vi "GDSProject_GetFullItemName.vi"(4 "error in (no error)":errorcluster, 7 "ProjectItem Refnum":refnum<vi>) -> (0 "error out":errorcluster, 3 "ItemFullName":string)   [LabVIEW 2020]
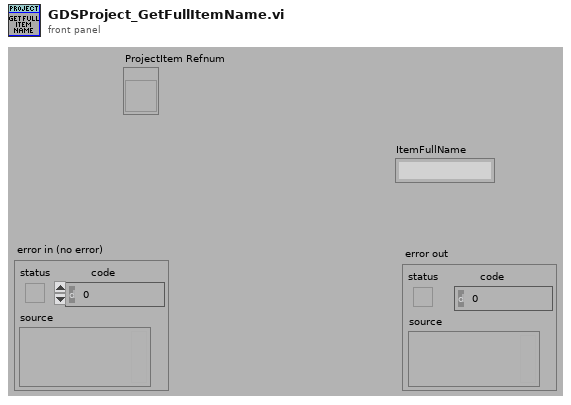
[diagram p1: front panel]
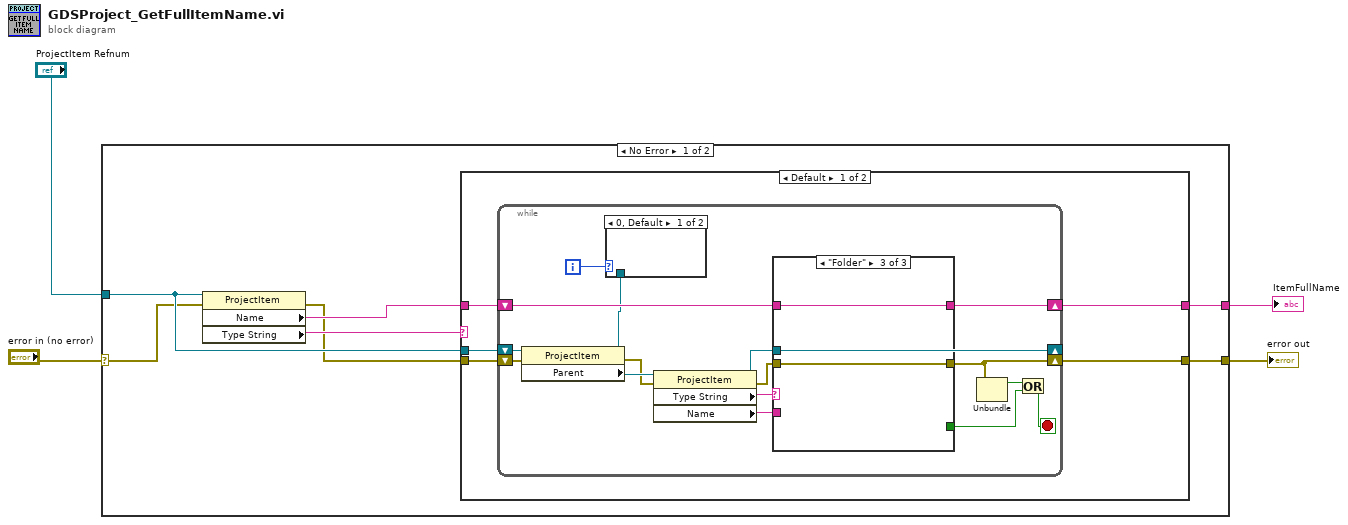
[diagram p0: block diagram]
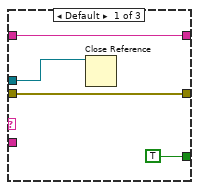
[diagram p2: hidden frame]
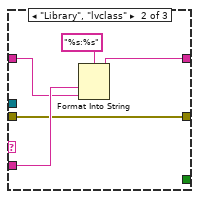
[diagram p3: hidden frame]
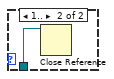
[diagram p4: hidden frame]
diagram:
  n1 = case shown="No Error" "error in (no error)" {
    selector: "error in (no error)" -> [w6 w46]
    tunnel: [w8 w46] -> w2
    tunnel: "ProjectItem Refnum" -> [w11 _]
    tunnel: [w7 _] -> w1
    frame No Error {
      n2 = property class="ProjectItem"(reference=w11, error in=w6) -> (error out=w5:errorcluster, "Name"=w9:string, "Type String"=w10:string)  [unwired: 1 out]
      n3 = case shown="Default" w10 {
        tunnel: w11 -> [w16 _]
        tunnel: w9 -> [w15 _]
        tunnel: w5 -> [w14 w45]
        tunnel: [w13 w45] -> w8
        tunnel: [w12 _] -> w7
        frame Default {
          n4 = while {
            shift-right: [w17] -> _
            shift-left: w16 -> [w32]
            shift-right: [w20] -> w12
            shift-left: w15 -> [w21]
            shift-right: [w26] -> w13
            shift-left: w14 -> [w27]
            i -> [w31]
            stop <- w23 stop-if-true
            n5 = property class="ProjectItem"(reference=w32, error in=w27) -> (reference out=w18:refnum<vi>, error out=w19:errorcluster, "Parent"=w30:refnum<vi>)
            n6 = case shown="0, Default" w31 {
              tunnel: w18 -> [_ w44]
              frame 0, Default {
              }
              frame 1.. {
                n7 = Close Reference(reference=w44) -> ()  [unwired: 1 in, 1 out]
              }
            }
            n8 = property class="ProjectItem"(reference=w30, error in=w19) -> (reference out=w17:refnum<vi>, error out=w28:errorcluster, "Type String"=w29:string, "Name"=w22:string)
            n9 = case shown="\"Folder\"" w29 {
              tunnel: [w36 w37 w43] -> w26
              tunnel: w28 -> [w36 w37 w43]
              tunnel: [TRUE _ _] -> w24
              tunnel: w22 -> [_ w40 _]
              tunnel: w21 -> [w34 w39 w42]
              tunnel: [w34 w38 w42] -> w20
              tunnel: w17 -> [w33 _ _]
              frame Default {
                n10 = Close Reference(reference=w33) -> ()  [unwired: 1 in, 1 out]
              }
              frame "Library", "lvclass" {
                n11 = Format Into String(format string="%s:%s", w40, w39) -> (resulting string=w38:string)  [unwired: 2 in, 1 out]
              }
              frame "Folder" {
              }
            }
            n12 = Unbundle(w26) -> ("status"=w25:bool)  [unwired: 2 out]
            n13 = Or(x=w25, y=w24) -> (x .or. y?=w23:bool)
          }
        }
        frame "Folder" {
        }
      }
    }
    frame Error {
    }
  }
  "ItemFullName" <- w1
  "error out" <- w2
